vi "Init Hardware.vi"(8 "error in (no error)":errorcluster, 11 "Temperature Controller Driver in":refnum<class "Temperature Controller Driver.lvclass">) -> (0 "error out":errorcluster, 3 "Temperature Controller Driver out":refnum<class "Temperature Controller Driver.lvclass">)   [LabVIEW 2019, in "Temperature Controller Driver.lvclass"]
uses:
  Temperature Controller Driver.lvclass
  C:/GitHub/NHMFL_Core/Libraries/Instruments/Instrument Driver/Instrument Driver.lvclass
  Instrument Driver/Instrument Driver.lvclass/Instrument Driver.ctl
  Instrument Driver/Read Recorder name.vi
  Instrument Driver/Write Channel names.vi
  Instrument Driver/Write Channel units.vi
  Read T controller configuration.vi
  Simple VISA Reader/Simple VISA Reader Driver.lvclass
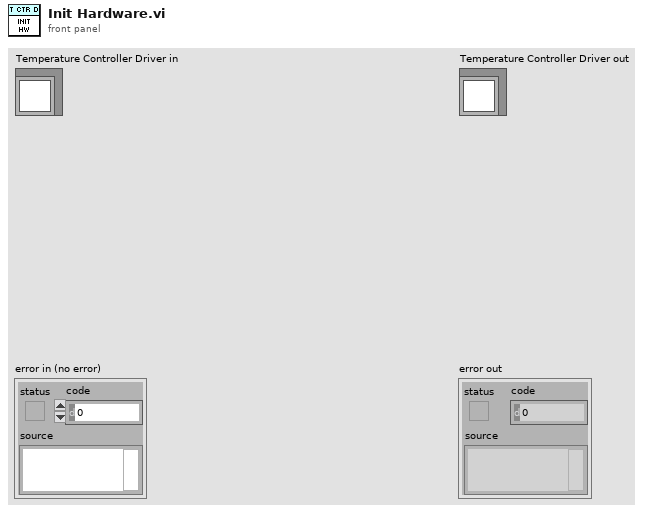
[diagram p1: front panel]
types:
  T1 = typedef "T controller configuration.ctl" = cluster{"Record Channels":string[], "Add raw signal":bool, "New set point":dbl, "Record heater":bool}
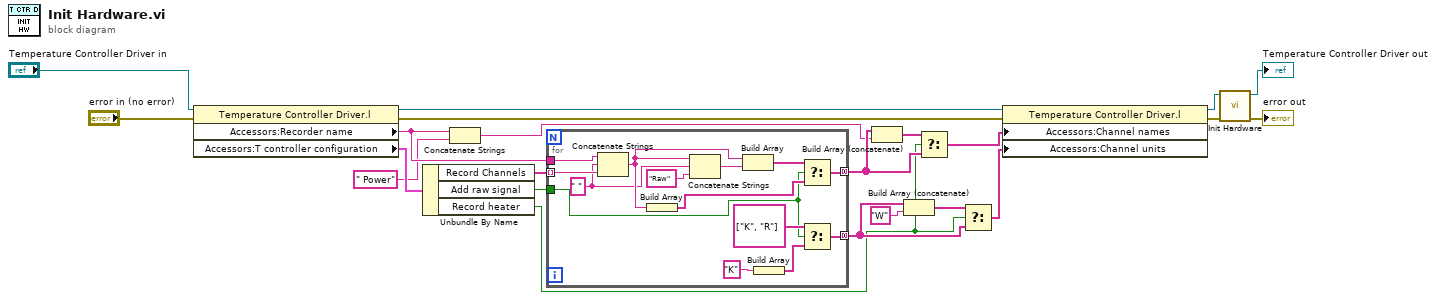
[diagram p0: block diagram]
diagram:
  n1 = property class="Temperature Controller Driver.l"(reference="Temperature Controller Driver in", error in="error in (no error)") -> (reference out=w19:refnum<class "Temperature Controller Driver.lvclass">, error out=w20:errorcluster, "Accessors:Recorder name"=w6:string, "Accessors:T controller configuration"=w16:T1)
  n2 = Unbundle By Name(w16) -> ("Record Channels"=w15:string[], "Add raw signal"=w14:bool, "Record heater"=w2:bool)
  n3 = Concatenate Strings(w6, " Power" ("string")) -> (w3:string)
  n4 = for {
    tunnel: w15 -> [w35] mode=indexing
    tunnel: w14 -> [w27]
    tunnel: [w24] -> w4 mode=concatenating
    tunnel: [w23] -> w9 mode=concatenating
    tunnel: w6 -> [w36]
    w25 = " "
    n5 = Concatenate Strings(w36, w25, w35) -> (w26:string)
    n6 = Build Array(w26) -> (w31:string[])
    n7 = Concatenate Strings(w26, w25, "Raw" ("string")) -> (w33:string)
    n8 = Build Array(w26, w33) -> (w32:string[])
    n9 = Build Array("K") -> (w29:string[])
    n10 = Select(t=w32, s=w27, f=w31) -> (s? t:f=w24:string[])
    n11 = Select(t=string[] ["K", "R"], s=w27, f=w29) -> (s? t:f=w23:string[])
  }
  n12 = Build Array (concatenate)(w4, w3) -> (w7:string[])
  n13 = Build Array (concatenate)(w9, "W") -> (w11:string[])
  n14 = Select(t=w7, s=w2, f=w4) -> (s? t:f=w1:string[])
  n15 = Select(t=w11, s=w2, f=w9) -> (s? t:f=w8:string[])
  n16 = property class="Temperature Controller Driver.l"(reference=w19, error in=w20, "Accessors:Channel names"=w1, "Accessors:Channel units"=w8) -> (reference out=w17:refnum<class "Temperature Controller Driver.lvclass">, error out=w12:errorcluster)
  n17 = call-parent "Init Hardware.vi"("error in (no error)"=w12, "Instrument Driver in"=w17) -> ("error out"=→"error out":errorcluster, "Instrument Driver out"=→"Temperature Controller Driver out":refnum<class "Temperature Controller Driver.lvclass">)  [unwired: 8 in]
